vi "disable_ctrl.vi"(8 "Error in":errorcluster caption="Error in (no error)", 9 "disabled? (F)":bool, 10 "control name":string, 11 "vi ref":refnum<vi>) -> (0 "Error out":errorcluster, 3 "vi ref (duplicate)":refnum<vi>)   [LabVIEW 2015]
uses:
  polys/poly_control_ref_from_name_single.vi
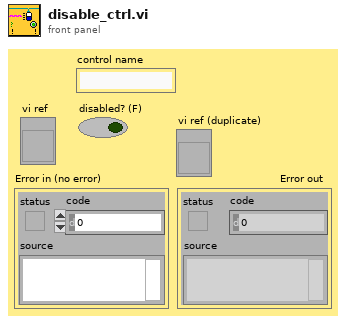
[diagram p1: front panel]
types:
  T1 = enum8{"Enabled", "Disabled", "Disabled and Grayed Out"}
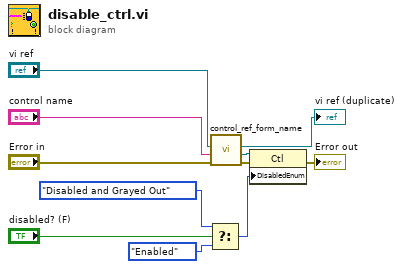
[diagram p0: block diagram]
diagram:
  n1 = Select(t=T1."Disabled and Grayed Out" ("Disabled"), s="disabled? (F)", f=T1."Enabled" ("Disabled")) -> (s? t:f=w11:T1)
  n2 = call-poly "control_ref_form_name.vi"("error in (no error)"="Error in", "control name"="control name", "vi ref"="vi ref") -> ("error out"=w1:errorcluster, "ctrl ref"=w4:refnum<vi>, "vi ref dup"=→"vi ref (duplicate)":refnum<vi>)  [unwired: 5 in, 1 out]
  n3 = property class="Ctl"(reference=w4, error in=w1, "DisabledEnum"=w11) -> (error out=→"Error out":errorcluster)  [unwired: 1 out]
